vi "1D Linear Evaluation (DBL).vi"(2 "b":dbl, 3 "a":dbl, 4 "X":dbl[](array[numeric])) -> (0 "error":i32, 1 "Y[i]=X[i]*a+b":dbl[](array[numeric]))   [LabVIEW 2020, in "NI_AALPro.lvlib"]
doc: "Performs a linear evaluation on every element of <B>X</B> using the scale <B>a</B> and the offset <B>b</B>. Wire data to the <B>X</B> input to determine the polymorphic instance to use or manually select the instance."
uses:
  <vilib>/Analysis/NI_AALPro.lvlib
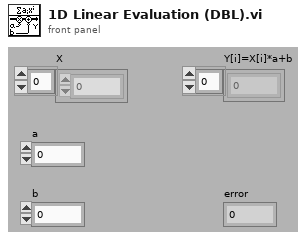
[diagram p1: front panel]
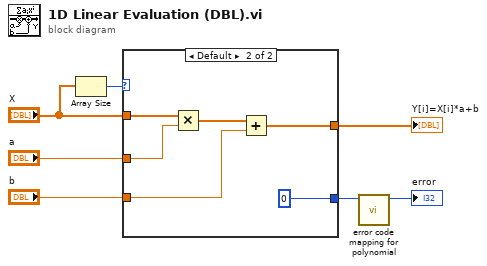
[diagram p0: block diagram]
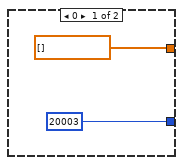
[diagram p2: hidden frame]
diagram:
  n1 = Array Size(array="X") -> (size(s)=w6:i32)
  n2 = case shown="Default" w6 {
    tunnel: "X" -> [_ w15]
    tunnel: "a" -> [_ w14]
    tunnel: "b" -> [_ w12]
    tunnel: [dbl[] [] w11] -> w3
    tunnel: [20003 ("empty array") 0] -> w2
    frame 0 {
    }
    frame Default {
      n3 = Multiply(x=w15, y=w14) -> (x*y=w13:dbl[])
      n4 = Add(x=w13, y=w12) -> (x+y=w11:dbl[])
    }
  }
  "Y[i]=X[i]*a+b" <- w3
  n5 = call <vilib>:"error code mapping for polynomial.vi"("error in"=w2) -> ("error out"=→"error":i32)  [unwired: 10 in]
